vi "LVH5AreadString.vi"(6 "error in (no error)":errorcluster, 8 "Name":string, 9 "HDF5 Location in":T1) -> (0 "error out":errorcluster, 1 "Value":string, 3 "HDF5 Location out":T1)   [LabVIEW 2017]
doc: "This is a high level VI for writing string attributes only. It should not normally need to be called by users of LVHDF5. They should instead call Simple H5Awrite. This was implemented to break a recursion cycle in Type Caching."
uses:
  <vilib>/UPVI/lvhdf5/library.llb/HDF5 Ref.ctl
  <vilib>/UPVI/lvhdf5/h5helper.dll
panel:
  # "LVHDF5 Toolkit\nCopyright (c) 2005-2013 by Jason D. Sommerville\nCopyright (c) 2014 by UPVI, LLC.\n\nThis use and distribution of this file is governed by the terms found in \nLICENSE.txt distributed with this toolkit and installed at\n <user.lib>\\_lvhdf5\\LICENSE.txt"
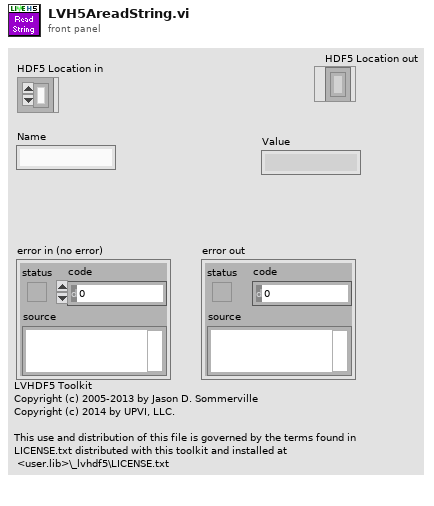
[diagram p1: front panel]
types:
  T1 = typedef "HDF5 Ref.ctl" = refnum<k1>
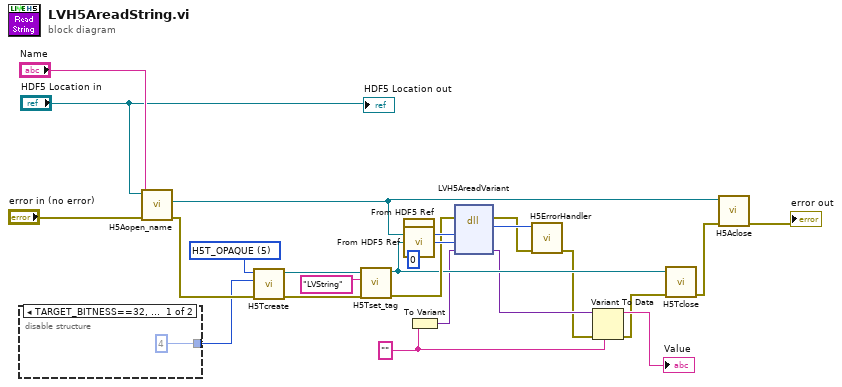
[diagram p0: block diagram]
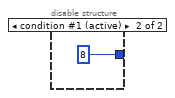
[diagram p2: hidden frame]
diagram:
  w4 = ""
  (unwired) 0 ("rank")
  w15 = 5 items=["H5T_NO_CLASS"=-1, "H5T_INTEGER"=0, "H5T_FLOAT"=1, "H5T_TIME"=2, "H5T_STRING"=3, "H5T_BITFIELD"=4, "H5T_OPAQUE"=5, "H5T_COMPOUND"=6, "H5T_REFERENCE"=7, "H5T_ENUM"=8, "H5T_VLEN"=9, "H5T_ARRAY"=10] ("class")
  n1 = disable-structure shown="TARGET_BITNESS==32, default" {
    disable-tunnel: [u32 4 ("size") u32 8 ("size")] -> w1
    frame condition #0 {
    }
    frame condition #1 (active) {
    }
  }
  n2 = call <vilib>:"H5Aopen_name.vi"("error in (no error)"="error in (no error)", "name"="Name", "HDF5 Ref"="HDF5 Location in") -> ("error out"=w21:errorcluster, "HDF5 Attr Ref"=w12:T1)  [unwired: 4 in, 1 out]
  n3 = call <vilib>:"H5Tcreate.vi"("error in (no error)"=w21, "size"=w1, "class"=w15) -> ("error out"=w18:errorcluster, "HDF5 Type Ref out"=w17:T1)  [unwired: 5 in]
  n4 = call <vilib>:"H5Tset_tag.vi"("error in (no error)"=w18, "Tag"="LVString" ("format string"), "HDF5 Ref"=w17) -> ("error out"=w22:errorcluster, "HDF5 Ref out"=w13:T1)  [unwired: 5 in]
  n5 = call <vilib>:"From HDF5 Ref.vi"("HDF5 Ref"=w12) -> ("I32"=w24:i32)
  n6 = call <vilib>:"From HDF5 Ref.vi"("HDF5 Ref"=w13) -> ("I32"=w23:i32)
  n7 = To Variant(anything=w4) -> (Variant=w8:variant)
  n8 = dll-call lib="C:/Program Files/National Instruments/LabVIEW 2017/vi.lib/UPVI/lvhdf5/h5helper.dll" fn="LVH5AreadVariant"(error in=w22, "attr_id"=w24, "mem_type_id"=w23, "Value"=w8) -> (error out=w6:errorcluster, "return type"=w14:i32, "Value"=w5:variant)  [unwired: 4 in, 1 out]
  n9 = call <vilib>:"H5ErrorHandler.vi"("error in (no error)"=w6, "herr_t"=w14) -> ("error out"=w3:errorcluster)  [unwired: 3 in, 4 out]
  n10 = Variant To Data(error in=w3, type=w4, Variant=w5) -> (data=→"Value":string, error out=w2:errorcluster)
  n11 = call <vilib>:"H5Tclose.vi"("error in (no error)"=w2, "HDF5 Datatype Ref"=w13) -> ("error out"=w11:errorcluster)  [unwired: 7 in]
  n12 = call <vilib>:"H5Aclose.vi"("error in (no error)"=w11, "HDF5 Dataset Ref"=w12) -> ("error out"=→"error out":errorcluster)  [unwired: 7 in]
  "HDF5 Location out" <- "HDF5 Location in"
